vi "Error handler.vi"(6 "error in (no error)":errorcluster, 7 "stop":bool, 8 "period (ms)":i64=10, 9 "emergency object in":refnum<k20>) -> (0 "error out":errorcluster, 1 "Is new?":bool, 3 "emergency object out":refnum<k20>, 4 "timestamp":timestamp)   [LabVIEW 2016]
uses:
  <vilib>/Platform/TimedLoop/XDataNode/timing_clust.ctl
  <vilib>/Platform/TimedLoop/XDataNode/nitl_modes.ctl
  <vilib>/Platform/TimedLoop/XDataNode/wakeup.ctl
  <vilib>/CANopenLib/CANOPEN.llb/CANopen Emergency Start.vi
  <vilib>/CANopenLib/CANOPEN.llb/CANopen Emergency Read.vi
  <vilib>/Platform/TimedLoop/XDataNode/XDataNode.xnode
  <vilib>/Platform/TimedLoop/XDataNode/XDNodeRunTimeDep.lvlib
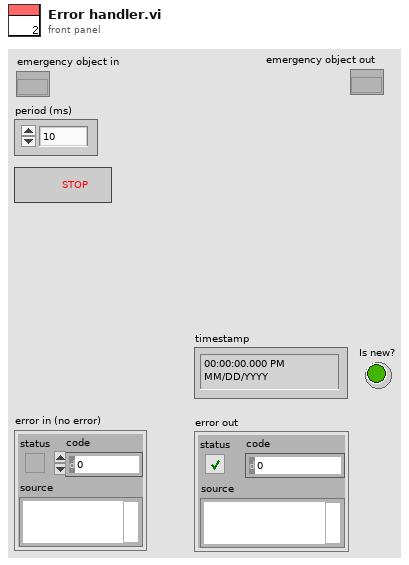
[diagram p1: front panel]
types:
  T1 = typedef "XDNodeRunTimeDep.lvlib/timing_clust.ctl" = cluster{"Expected End [f-1]":u64, "Actual End [f-1]":u64, "Finished Late? [f-1]":bool, "Expected End [i-1]":u64, "Actual End [i-1]":u64, "Finished Late? [i-1]":bool, "Expected Start [i]":u64, "Actual Start [i]":u64, "Expected Start [f]":u64, "Actual Start [f]":u64, "Source Name":string, "Structure Name":string, "Period":i64, "Deadline":i64, "Offset":i64, "Start":i64, "Priority":i32, "Timeout":i32, "Mode":T2, "Wakeup Reason":T3, "Error":errorcluster, "Source Type":string, "Secondary Source Type":string, "Global End Time":u64, "Global Start Time":u64, "Frame Duration":u64, "Iteration Duration":u64, "Assigned CPU":i32, "I/O Scan Engine Mode":u32}
  T2 = typedef "XDNodeRunTimeDep.lvlib/nitl_modes.ctl" = enum32{"No Change", "Process missed periods, maintain original phase", "Discard missed periods, maintain original phase", "Process missed periods, ignore original phase", "Discard missed periods, ignore original phase"}
  T3 = typedef "XDNodeRunTimeDep.lvlib/wakeup.ctl" = enum32{"Normal", "Aborted", "Asynchronous wakeup", "Timing source error", "Timed loop error", "Timeout"}
  T4 = cluster{"error code":u16, "error register":u8, "manufacturer specific error field":u8[]}
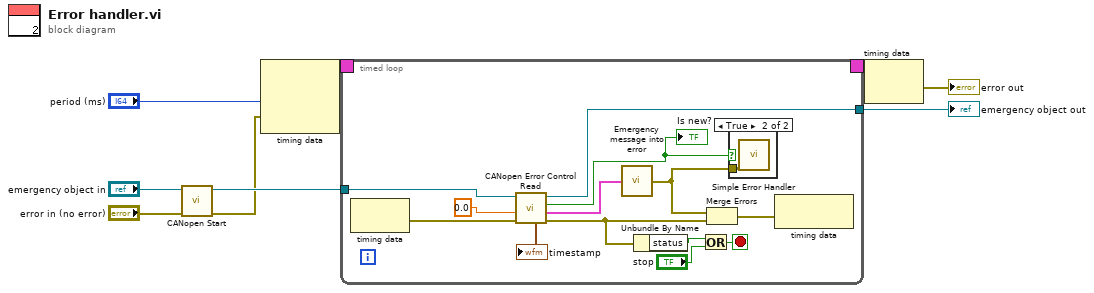
[diagram p0: block diagram]
diagram:
  n1 = call-poly <vilib>:"CANopen Start.vi"("error in (no error)"="error in (no error)", "emergency object in"="emergency object in") -> ("error out"=w5:errorcluster, "emergency object out"=w7:refnum<k20>)  [unwired: 8 in]
  n2 = node-c288("period (ms)", w5) -> (w9:T1)  [unwired: 1 in]
  n3 = timed-loop {
    tunnel: w7 -> [w21]
    tunnel: [w20] -> w1
    timing: w9 -> [_]
    timing-out: [_] -> w8
    stop <- w18 stop-if-true
    n4 = node-c288() -> (w15:errorcluster)  [unwired: 1 in]
    n5 = call-poly <vilib>:"CANopen Error Control Read.vi"("error in (no error)"=w15, "timeout (0s)"=0.0 ("timeout(0)"), "emergency object in"=w21) -> ("error out"=w13:errorcluster, "emergency message"=w14:T4, "new message?"=w11:bool, "emergency object out"=w20:refnum<k20>, "timestamp"=→"timestamp":timestamp)  [unwired: 4 in]
    "Is new?" <- w11
    n6 = call "Emergency message into error.vi"("emergency message"=w14) -> ("error"=w10:errorcluster)
    n7 = Unbundle By Name(w13) -> ("status"=w16:bool)
    n8 = Or(x=w16, y="stop") -> (x .or. y?=w18:bool)
    n9 = Merge Errors(w10, w13) -> (w12:errorcluster)
    n10 = case shown="True" w11 {
      tunnel: w10 -> [_ w23]
      frame False {
      }
      frame True {
        n11 = call <vilib>:"Simple Error Handler.vi"("error in (no error)"=w23) -> ()  [unwired: 4 in, 5 out]
      }
    }
    n12 = node-c288(w12) -> ()  [unwired: 1 out]
  }
  "emergency object out" <- w1
  n13 = node-c288(w8) -> (→"error out":errorcluster)
